vi "Write Test Step To UI.vi"(8 "error in (no error)":errorcluster, 11 "Step":i32) -> (0 "error out":errorcluster)   [LabVIEW 2015]
uses:
  User Interface/UI Handler/UI Handler.lvclass
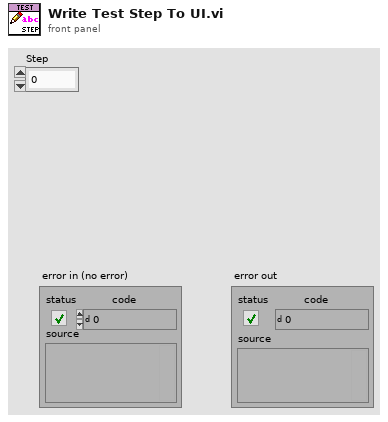
[diagram p1: front panel]
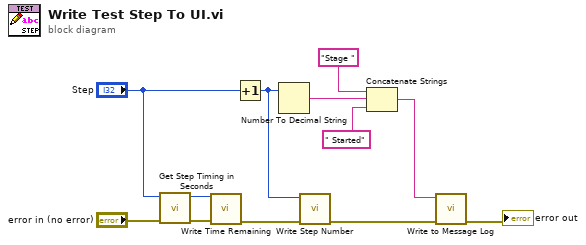
[diagram p0: block diagram]
diagram:
  n1 = call "Get Step Timing in Seconds.vi"("error in (no error)"="error in (no error)", "Step Index"="Step") -> ("error out"=w3:errorcluster, "Timing"=w1:i32)  [unwired: 8 in]
  n2 = call "Write Time Remaining.vi"("error in (no error)"=w3, "Value"=w1) -> ("error out"=w2:errorcluster)  [unwired: 9 in]
  n3 = Increment(x="Step") -> (x+1=w9:i32)
  n4 = Number To Decimal String(number=w9) -> (decimal integer string=w11:string)  [unwired: 1 in]
  n5 = call "Write Step Number.vi"("error in (no error)"=w2, "Value"=w9) -> ("error out"=w7:errorcluster)  [unwired: 9 in]
  n6 = Concatenate Strings("Stage " ("decimal integer string"), w11, " Started" ("string")) -> (w8:string)
  n7 = call "Write to Message Log.vi"("error in (no error)"=w7, "Message"=w8) -> ("error out"=→"error out":errorcluster)  [unwired: 9 in]
